vi "Compare Labels.vi"(9 "refresh listbox":T6[](array[typedef]), 10 "new label":T1, 11 "old label":T1) -> (1 "refresh listbox out":T6[](array[typedef]), 2 "any changes?":bool)   [LabVIEW 2020, in "Ballard ARINC 429 System Explorer.lvlib" / "Implementation.lvlib"]
uses:
  Implementation.lvlib
  Types/Refresh Listbox.ctl
  Types/Refresh Symbols.ctl
  Shared/VS Channels Definition for Label.ctl
  Shared/VS Channel Definition for Parameter.ctl
  Shared/Parameter Definition.ctl
  <vilib>/NI/NI VeriStand Encoding and Decoding/Encoding.ctl
  Shared/Transfer Type.ctl
  Refresh Constants.vi
  <vilib>/NI/NI VeriStand Encoding and Decoding/Encoding and Decoding.lvlib
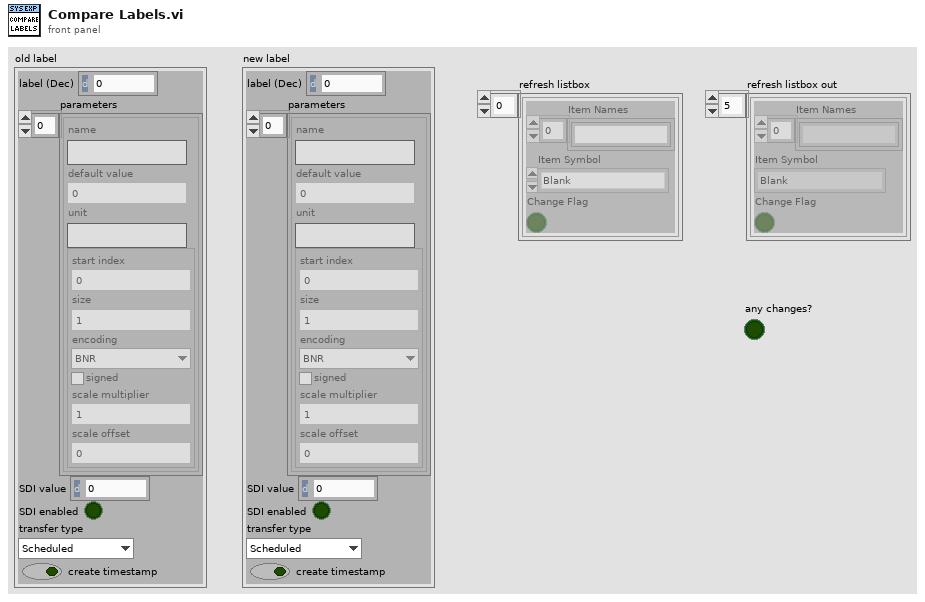
[diagram p1: front panel]
types:
  T1 = typedef "VS Channels Definition for Label.ctl" = cluster{"label (Dec)":u32, "parameters":T2[], "SDI value":u8, "SDI enabled":bool, "transfer type":T5, "create timestamp":bool}
  T2 = typedef "VS Channel Definition for Parameter.ctl" = cluster{"name":string, "default value":dbl, "unit":string, "Parameter":T3}
  T3 = typedef "Parameter Definition.ctl" = cluster{"start index":i32, "size":i32, "encoding":T4, "signed":bool, "scale multiplier":dbl, "scale offset":dbl}
  T4 = typedef "Encoding and Decoding.lvlib/Encoding.ctl" = enum16{"BNR", "BCD", "Discrete"}
  T5 = typedef "Transfer Type.ctl" = enum16{"Scheduled", "Acyclic", "Block", "Strobe"}
  T6 = typedef "Ballard ARINC 429 System Explorer.lvlib/Implementation.lvlib/Refresh Listbox.ctl" = cluster{"Item Names":string[], "Item Symbol":T7, "Change Flag":bool}
  T7 = typedef "Ballard ARINC 429 System Explorer.lvlib/Implementation.lvlib/Refresh Symbols.ctl" = enum16{"Blank", "Port", "Incoming", "Outgoing", "Label", "Word", "Parameter", "ARINC-429", "Config Files", "Channel Spec", "Item"}
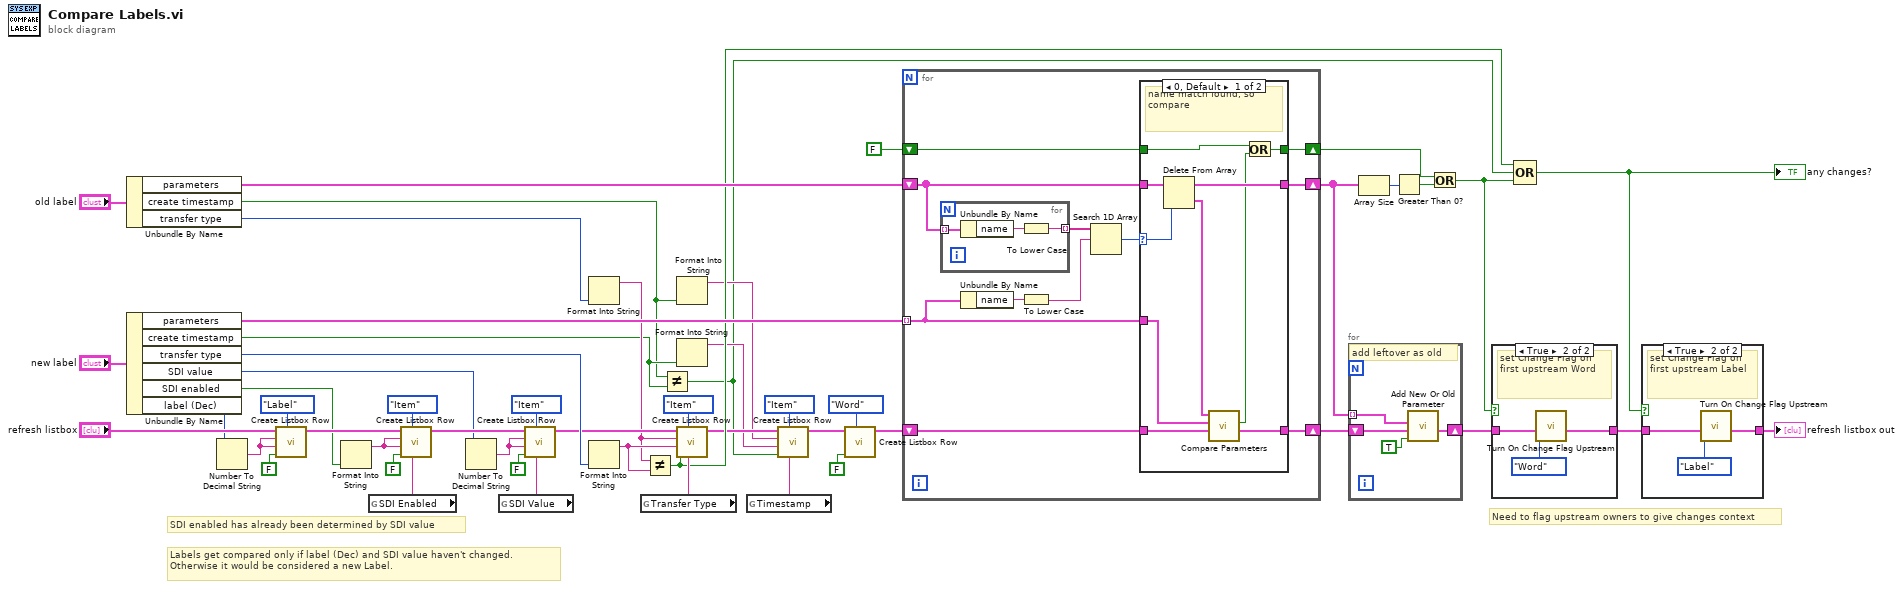
[diagram p0: block diagram]
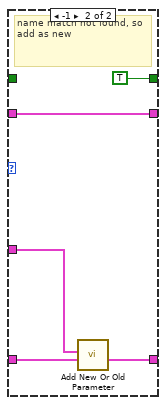
[diagram p4: hidden frame]
diagram:
  # "Labels get compared only if label (Dec) and SDI value haven't changed. Otherwise it would be considered a new Label."
  # "Need to flag upstream owners to give changes context"
  # "SDI enabled has already been determined by SDI value"
  n1 = Unbundle By Name("old label") -> ("parameters"=w29:T2[], "create timestamp"=w3:bool, "transfer type"=w33:T5)
  n2 = Unbundle By Name("new label") -> ("parameters"=w41:T2[], "create timestamp"=w4:bool, "transfer type"=w43:T5, "SDI value"=w46:u8, "SDI enabled"=w23:bool, "label (Dec)"=w50:u32)
  n3 = Number To Decimal String(number=w50) -> (decimal integer string=w36:string)  [unwired: 1 in]
  n4 = call "Create Listbox Row.vi"("refresh symbol (Blank)"=Refresh_Symbols."Label" ("Refresh Symbol (Blank)"), "change? (T)"=FALSE, "new item"=w36, "old item"=w36, "refresh listbox"="refresh listbox") -> ("refresh listbox out"=w48:T6[])  [unwired: 6 in]
  n5 = Format Into String(w23) -> (resulting string=w11:string)  [unwired: 3 in, 1 out]
  n6 = global read "Refresh Constants.vi" "SDI Enabled"() -> (w27:string)
  n7 = call "Create Listbox Row.vi"("override name"=w27, "refresh symbol (Blank)"=Refresh_Symbols."Item" ("Refresh Symbol (Blank)"), "change? (T)"=FALSE, "new item"=w11, "old item"=w11, "refresh listbox"=w48) -> ("refresh listbox out"=w47:T6[])  [unwired: 5 in]
  n8 = Number To Decimal String(number=w46) -> (decimal integer string=w34:string)  [unwired: 1 in]
  n9 = global read "Refresh Constants.vi" "SDI Value"() -> (w25:string)
  n10 = call "Create Listbox Row.vi"("override name"=w25, "refresh symbol (Blank)"=Refresh_Symbols."Item" ("Refresh Symbol (Blank)"), "change? (T)"=FALSE, "new item"=w34, "old item"=w34, "refresh listbox"=w47) -> ("refresh listbox out"=w42:T6[])  [unwired: 5 in]
  n11 = Format Into String(w33) -> (resulting string=w30:string)  [unwired: 3 in, 1 out]
  n12 = Format Into String(w43) -> (resulting string=w31:string)  [unwired: 3 in, 1 out]
  n13 = global read "Refresh Constants.vi" "Transfer Type"() -> (w26:string)
  n14 = Not Equal?(x=w30, y=w31) -> (x != y?=w12:bool)
  n15 = Not Equal?(x=w3, y=w4) -> (x != y?=w1:bool)
  n16 = Format Into String(w3) -> (resulting string=w6:string)  [unwired: 3 in, 1 out]
  n17 = Format Into String(w4) -> (resulting string=w5:string)  [unwired: 3 in, 1 out]
  n18 = call "Create Listbox Row.vi"("override name"=w26, "refresh symbol (Blank)"=Refresh_Symbols."Item" ("Refresh Symbol (Blank)"), "change? (T)"=w12, "new item"=w31, "old item"=w30, "refresh listbox"=w42) -> ("refresh listbox out"=w8:T6[])  [unwired: 5 in]
  n19 = global read "Refresh Constants.vi" "Timestamp"() -> (w2:string)
  n20 = call "Create Listbox Row.vi"("override name"=w2, "refresh symbol (Blank)"=Refresh_Symbols."Item" ("Refresh Symbol (Blank)"), "change? (T)"=w1, "new item"=w5, "old item"=w6, "refresh listbox"=w8) -> ("refresh listbox out"=w7:T6[])  [unwired: 5 in]
  n21 = call "Create Listbox Row.vi"("refresh symbol (Blank)"=Refresh_Symbols."Word" ("Refresh Symbol (Blank)"), "change? (T)"=FALSE, "refresh listbox"=w7) -> ("refresh listbox out"=w39:T6[])  [unwired: 8 in]
  n22 = for {
    shift-right: [w62] -> w24
    shift-left: w39 -> [w63]
    tunnel: w41 -> [w61] mode=indexing
    shift-right: [w55] -> w21
    shift-left: w29 -> [w56]
    shift-right: [w53] -> w18
    shift-left: FALSE -> [w54]
    n23 = for {
      tunnel: w56 -> [w80] mode=indexing
      tunnel: [w79] -> w59 mode=indexing
      n24 = Unbundle By Name(w80) -> ("name"=w81:string)
      n25 = To Lower Case(string=w81) -> (all lower case string=w79:string)
    }
    n26 = Unbundle By Name(w61) -> ("name"=w60:string)
    n27 = To Lower Case(string=w60) -> (all lower case string=w58:string)
    n28 = Search 1D Array(1D array=w59, element=w58) -> (index of element=w57:i32)  [unwired: 1 in]
    n29 = case shown="0, Default" w57 {
      selector: w57 -> [w72 _]
      tunnel: w63 -> [w69 w78]
      tunnel: [w70 w76] -> w62
      tunnel: w61 -> [w68 w77]
      tunnel: [w71 w75] -> w55
      tunnel: w56 -> [w73 w75]
      tunnel: w54 -> [w65 _]
      tunnel: [w66 TRUE] -> w53
      frame 0, Default {
        # "name match found, so compare"
        n30 = Delete From Array(array=w73, index=w72) -> (deleted portion=w67:T2, array with subset deleted=w71:T2[])  [unwired: 1 in]
        n31 = call "Compare Parameters.vi"("refresh listbox"=w69, "new parameter"=w68, "old parameter"=w67) -> ("refresh listbox out"=w70:T6[], "any changes?"=w64:bool)  [unwired: 7 in]
        n32 = Or(x=w65, y=w64) -> (x .or. y?=w66:bool)
      }
      frame -1 {
        # "name match not found, so add as new"
        n33 = call "Add New Or Old Parameter.vi"("refresh listbox"=w78, "channel parameter"=w77) -> ("refresh listbox out"=w76:T6[])  [unwired: 9 in]
      }
    }
  }
  n34 = for {
    shift-right: [w83] -> w17
    shift-left: w24 -> [w85]
    tunnel: w21 -> [w82] mode=indexing
    # "add leftover as old"
    n35 = call "Add New Or Old Parameter.vi"("old port?"=TRUE, "refresh listbox"=w85, "channel parameter"=w82) -> ("refresh listbox out"=w83:T6[])  [unwired: 8 in]
  }
  n36 = Array Size(array=w21) -> (size(s)=w20:i32)
  n37 = Greater Than 0?(x=w20) -> (x > 0?=w19:bool)
  n38 = Or(x=w18, y=w19) -> (x .or. y?=w16:bool)
  n39 = case shown="True" w16 {
    tunnel: w17 -> [w86 w89]
    tunnel: [w86 w87] -> w15
    frame False {
    }
    frame True {
      # "set Change Flag on first upstream Word"
      n40 = call "Turn On Change Flag Upstream.vi"("symbol to change"=Refresh_Symbols."Word", "refresh listbox"=w89) -> ("refresh listbox out"=w87:T6[])  [unwired: 9 in]
    }
  }
  n41 = Compound Arithmetic op=OR(w12, w1, w16) -> (w14:bool)
  "any changes?" <- w14
  n42 = case shown="True" w14 {
    tunnel: w15 -> [w90 w91]
    tunnel: [w90 w92] -> w13
    frame False {
    }
    frame True {
      # "set Change Flag on first upstream Label"
      n43 = call "Turn On Change Flag Upstream.vi"("symbol to change"=Refresh_Symbols."Label", "refresh listbox"=w91) -> ("refresh listbox out"=w92:T6[])  [unwired: 9 in]
    }
  }
  "refresh listbox out" <- w13
